vi "4_4.vi"() -> ()   [LabVIEW 2012]
panel:
  in  "stop":bool
  in  "OK Button":bool
  out "Numeric":dbl
  in  "а":dbl
  in  "б":dbl
  in  "Slide":i32(slide) scale=0.0..3.0
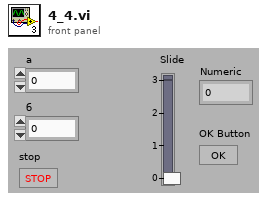
[diagram p1: front panel]
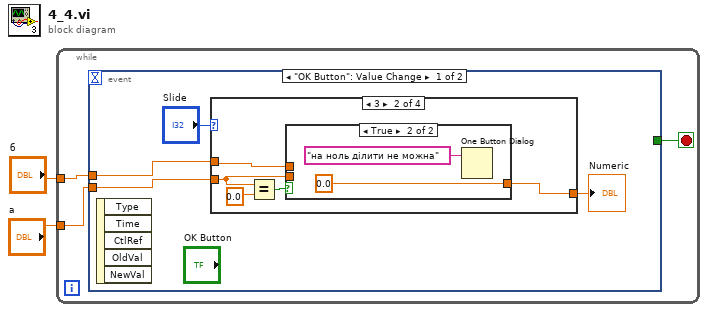
[diagram p0: block diagram]
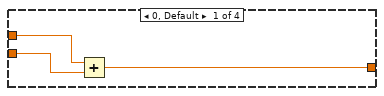
[diagram p2: hidden frame]
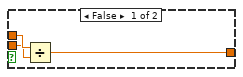
[diagram p3: hidden frame]
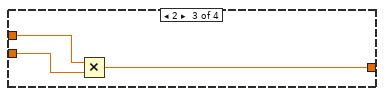
[diagram p4: hidden frame]
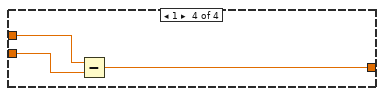
[diagram p5: hidden frame]
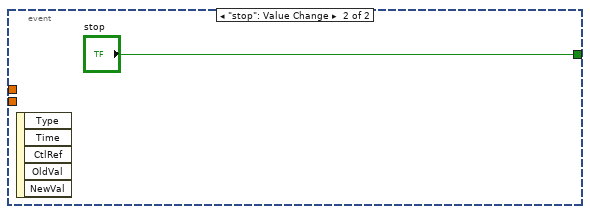
[diagram p6: hidden frame]
diagram:
  n1 = while {
    tunnel: "б" -> [w5]
    tunnel: "а" -> [w4]
    stop <- w3 stop-if-true
    n2 = event shown="[0] \"OK Button\": Value Change" {
      selector: _ -> [_ _]
      dyn-events: _ -> [_ _]
      timeout: _ -> [_ _]
      tunnel: w5 -> [w9 _]
      tunnel: w4 -> [w8 _]
      tunnel: [_ "stop"] -> w3
      event "OK Button": Value Change {
        n3 = event-data() -> ()  [unwired: 1 in, 5 out]
        n4 = case shown="3" "Slide" {
          tunnel: w9 -> [w12 w15 w25 w28]
          tunnel: w8 -> [w11 w13 w24 w27]
          tunnel: [w10 w14 w23 w26] -> w7
          frame 0, Default {
            n5 = Add(x=w12, y=w11) -> (x+y=w10:dbl)
          }
          frame 3 {
            n6 = Equal?(x=w13, y=0.0) -> (x = y?=w16:bool)
            n7 = case shown="True" w16 {
              tunnel: w15 -> [w20 _]
              tunnel: [w19 0.0] -> w14
              tunnel: w13 -> [w18 _]
              frame False {
                n8 = Divide(x=w20, y=w18) -> (x/y=w19:dbl)
              }
              frame True {
                n9 = One Button Dialog(message="на ноль ділити не можна") -> ()  [unwired: 1 in, 1 out]
              }
            }
          }
          frame 2 {
            n10 = Multiply(x=w25, y=w24) -> (x*y=w23:dbl)
          }
          frame 1 {
            n11 = Subtract(x=w28, y=w27) -> (x-y=w26:dbl)
          }
        }
        "Numeric" <- w7
      }
      event "stop": Value Change {
        n12 = event-data() -> ()  [unwired: 1 in, 5 out]
      }
    }
  }
